vi "Write Data.vi"(8 "error in (no error)":errorcluster, 10 "Base Data Lib:Data":refnum<class "Data.lvclass">, 11 "File Data Message in":refnum<class "File Data Message.lvclass">) -> (0 "error out":errorcluster, 3 "File Data Message out":refnum<class "File Data Message.lvclass">)   [LabVIEW 2014, in "File Library.lvlib" / "File Data Message.lvclass"]
uses:
  File Data Message.lvclass
  reusable/Data/Data.lvclass
  File Data Message.lvclass/File Data Message.ctl
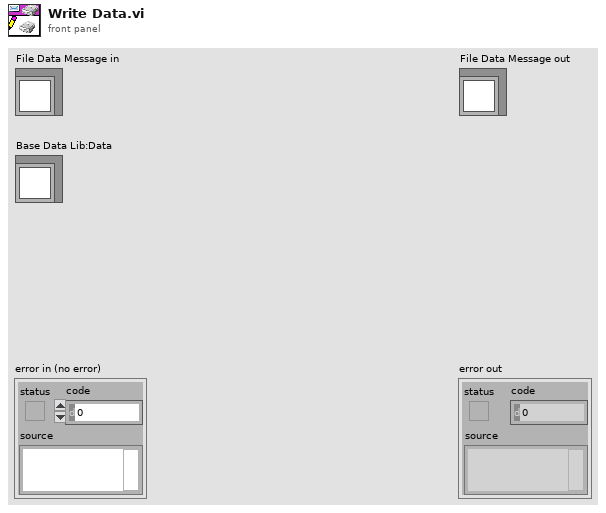
[diagram p1: front panel]
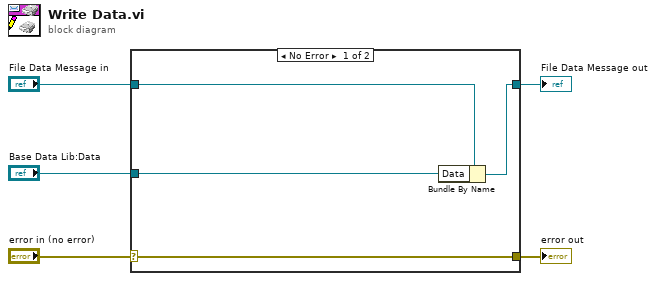
[diagram p0: block diagram]
diagram:
  n1 = case shown="No Error" "error in (no error)" {
    selector: "error in (no error)" -> [w9 w10]
    tunnel: [w9 w10] -> w4
    tunnel: [w7 w11] -> w2
    tunnel: "File Data Message in" -> [w8 w11]
    tunnel: "Base Data Lib:Data" -> [w6 _]
    frame No Error {
      n2 = Bundle By Name(cluster=w8, "Data"=w6) -> (w7:refnum<class "File Data Message.lvclass">)
    }
    frame Error {
    }
  }
  "error out" <- w4
  "File Data Message out" <- w2
